vi "X.1 PID.vi"(9 "2.1 PID Gains":T1={"P Gain"=0.25, "I Gain"=0.9999923706054688, "D Gain"=0.0, "P Gain - Exp"=2, "I Gain - Exp"=2, "D Gain - Exp"=2, "I Saturate"=0.25} {"I Saturate" format="%#_14g"; "P Gain" format="%.8f"; "I Gain" format="%.8f"; "D Gain" format="%.8f"}, 10 "Setpoint":i32, 11 "Encoder Value":i32) -> (0 "D Error":fxp<+/-,18,1> format="%.18g", 1 "I Error":fxp<+/-,64,46> format="%.32g", 2 "Analog Output":fxp<+/-,20,5> format="%.17g", 4 "Error":fxp<+/-,18,1> format="%.18g")   [LabVIEW 2010]
doc: "PID controll for FPGA (fixed point math) without the \"I\" or the \"D\""
uses:
  2-Low Neurons/2.1 PID Gains Typedef.ctl
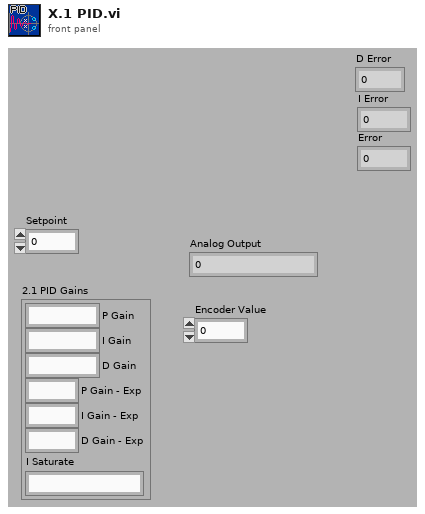
[diagram p1: front panel]
types:
  T1 = typedef "2.1 PID Gains Typedef.ctl" = cluster{"P Gain":fxp<+/-,18,1>, "I Gain":fxp<+/-,18,1>, "D Gain":fxp<+/-,18,1>, "P Gain - Exp":i8, "I Gain - Exp":i8, "D Gain - Exp":i8, "I Saturate":fxp<+/-,64,46>}
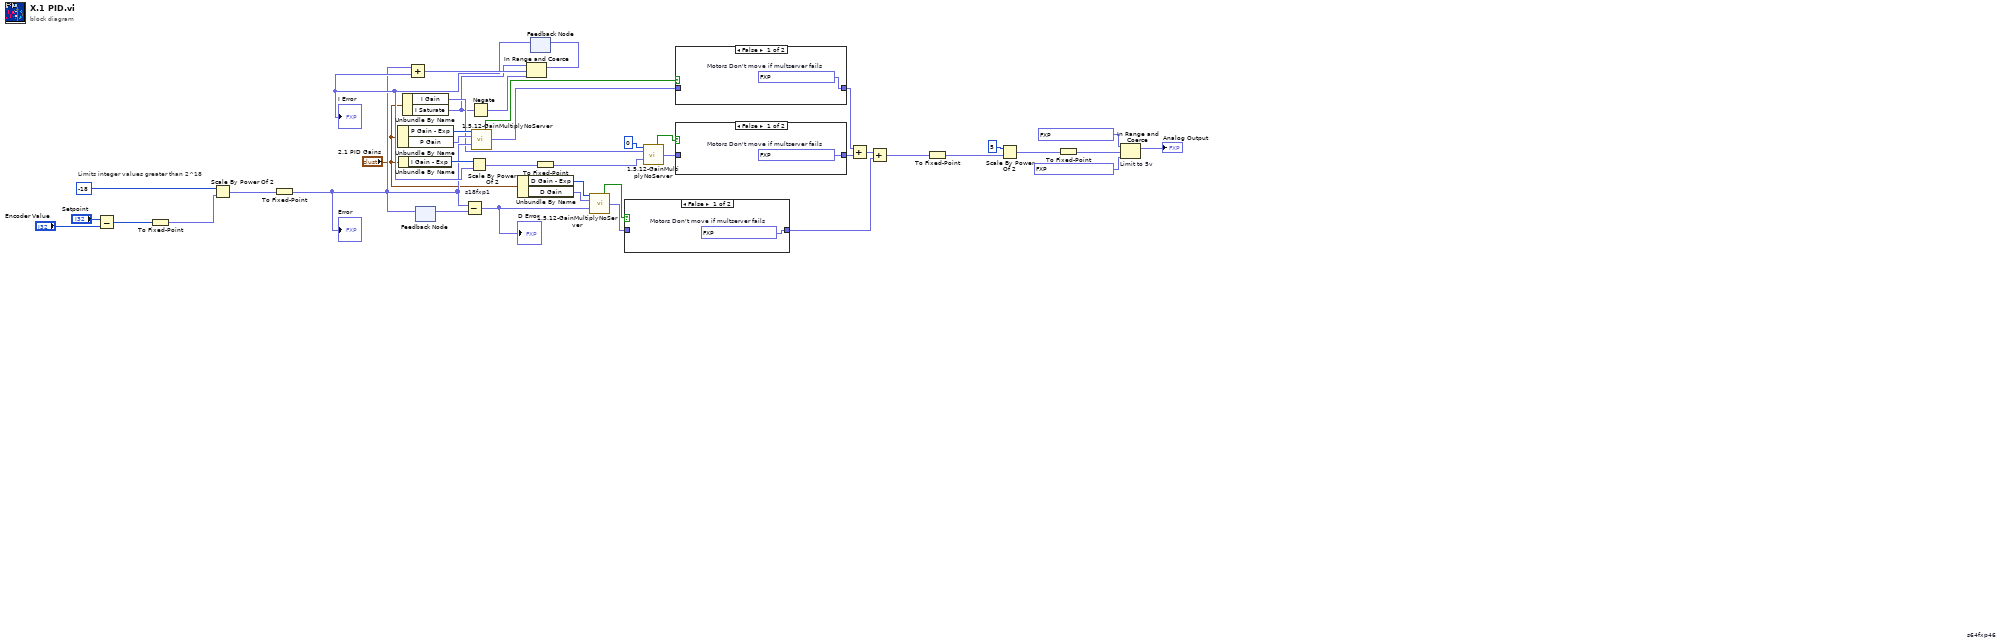
[diagram p0: block diagram]
diagram:
  # "Limits integer values greater than 2^18"
  n1 = Subtract(x="Setpoint", y="Encoder Value") -> (x-y=w39:i32)
  n2 = To Fixed-Point(number=w39) -> (fixed-point=w38:fxp<+/-,34,18>)  [unwired: 1 in]
  n3 = Scale By Power Of 2(n=-18, x=w38) -> (x*2^n=w37:fxp<+/-,34,18>)
  n4 = To Fixed-Point(number=w37) -> (fixed-point=w17:fxp<+/-,18,1>)  [unwired: 1 in]
  "Error" <- w17
  n5 = Unbundle By Name("2.1 PID Gains") -> ("P Gain - Exp"=w11:i8, "P Gain"=w12:fxp<+/-,18,1>)
  n6 = Unbundle By Name("2.1 PID Gains") -> ("I Gain - Exp"=w19:i8)
  n7 = Unbundle By Name("2.1 PID Gains") -> ("I Gain"=w10:fxp<+/-,18,1>, "I Saturate"=w2:fxp<+/-,64,46>)
  n8 = feedback-in #1(w17) -> ()
  n9 = feedback #1() -> (w16:fxp<+/-,18,1>)  [unwired: 1 in]
  n10 = Subtract "s18fxp1"(x=w17, y=w16) -> (x-y=w15:fxp<+/-,18,1>)
  "D Error" <- w15
  n11 = Negate(x=w2) -> (-x=w1:fxp<+/-,64,46>)
  n12 = call "1.5.12-GainMultiplyNoServer.vi"("Gain Exponent"=w11, "Gain"=w12, "Input"=w17) -> ("Result is Good"=w34:bool, "Output"=w33:fxp<+/-,18,1>)  [unwired: 11 in]
  n13 = Unbundle By Name("2.1 PID Gains") -> ("D Gain - Exp"=w8:i8, "D Gain"=w9:fxp<+/-,18,1>)
  n14 = feedback #2 "s64fxp46"() -> (w20:fxp<+/-,64,46>)  [unwired: 1 in]
  "I Error" <- w20
  n15 = Add(x=w17, y=w20) -> (x+y=w21:fxp<+/-,64,46>)
  n16 = Scale By Power Of 2(n=w19, x=w20) -> (x*2^n=w32:fxp<+/-,64,46>)
  n17 = In Range and Coerce(upper limit=w2, x=w21, lower limit=w1) -> (coerced(x)=w3:fxp<+/-,64,46>)  [unwired: 1 out]
  n18 = feedback-in #2(w3) -> ()
  n19 = To Fixed-Point(number=w32) -> (fixed-point=w31:fxp<+/-,18,1>)  [unwired: 1 in]
  n20 = call "1.5.12-GainMultiplyNoServer.vi"("Gain Exponent"=w8, "Gain"=w9, "Input"=w15) -> ("Result is Good"=w27:bool, "Output"=w30:fxp<+/-,18,1>)  [unwired: 11 in]
  n21 = case shown="False" w27 {
    tunnel: w30 -> [_ w44]
    tunnel: [w43 w44] -> w23
    frame False {
      w43 = fxp<+/-,18,1> 0.0  # Motors Don't move if multserver fails
    }
    frame True {
    }
  }
  n22 = call "1.5.12-GainMultiplyNoServer.vi"("Gain Exponent"=i8 0, "Gain"=w10, "Input"=w31) -> ("Result is Good"=w28:bool, "Output"=w29:fxp<+/-,18,1>)  [unwired: 11 in]
  n23 = case shown="False" w34 {
    tunnel: w33 -> [_ w46]
    tunnel: [w45 w46] -> w26
    frame False {
      w45 = fxp<+/-,18,1> 0.0  # Motors Don't move if multserver fails
    }
    frame True {
    }
  }
  n24 = case shown="False" w28 {
    tunnel: w29 -> [_ w48]
    tunnel: [w47 w48] -> w25
    frame False {
      w47 = fxp<+/-,18,1> 0.0  # Motors Don't move if multserver fails
    }
    frame True {
    }
  }
  n25 = Add(x=w26, y=w25) -> (x+y=w24:fxp<+/-,18,1>)
  n26 = Add(x=w24, y=w23) -> (x+y=w22:fxp<+/-,18,1>)
  n27 = To Fixed-Point(number=w22) -> (fixed-point=w7:fxp<+/-,23,6>)  [unwired: 1 in]
  n28 = Scale By Power Of 2(n=5, x=w7) -> (x*2^n=w6:fxp<+/-,23,6>)
  n29 = To Fixed-Point(number=w6) -> (fixed-point=w4:fxp<+/-,20,5>)  [unwired: 1 in]
  n30 = In Range and Coerce "Limit to 5v"(upper limit=fxp<+/-,20,5> 5.0, x=w4, lower limit=fxp<+/-,20,5> -5.0 ("upper limit")) -> (coerced(x)=→"Analog Output":fxp<+/-,20,5>)  [unwired: 1 out]
